vi "FTW-ProjectItemManager-Write-Session.vi"(0 "Project Item Manager":refnum<class "FTW-ProjectItemManager.lvclass">, 5 "Tag":string, 7 "Value":variant, 11 "error in":errorcluster) -> (4 "Project Item Manager out":refnum<class "FTW-ProjectItemManager.lvclass">, 15 "error out":errorcluster)   [LabVIEW 2012, in "FTW-ProjectItemManager.lvclass"]
doc: "This VI bypasses the Transaction Queue by writing a property directly to the Deploy Build Spec Project Item. The property is then persisted to disk if the user saves the LVProj, or if it is programmatically saved."
uses:
  FTW-ProjectItemManager.lvclass
  FTW-ProjectItemManager.lvclass/FTW-ProjectItemManager.ctl
panel:
  # "Inputs"
  # "Outputs"
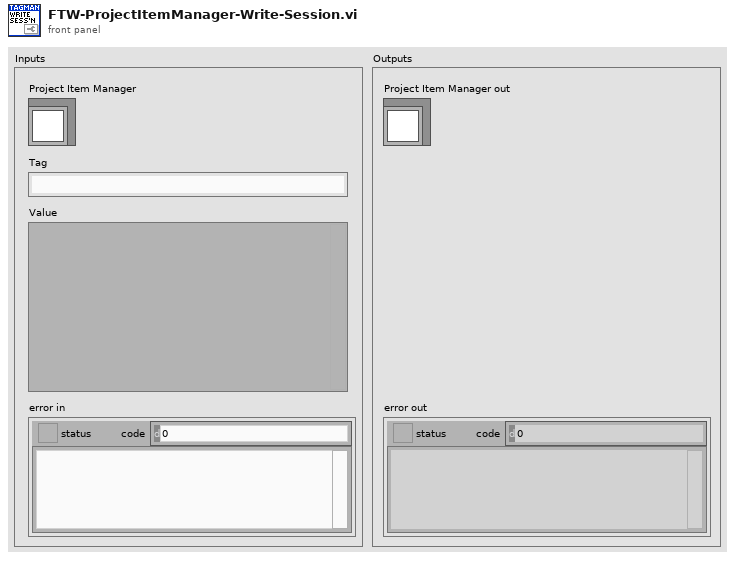
[diagram p1: front panel]
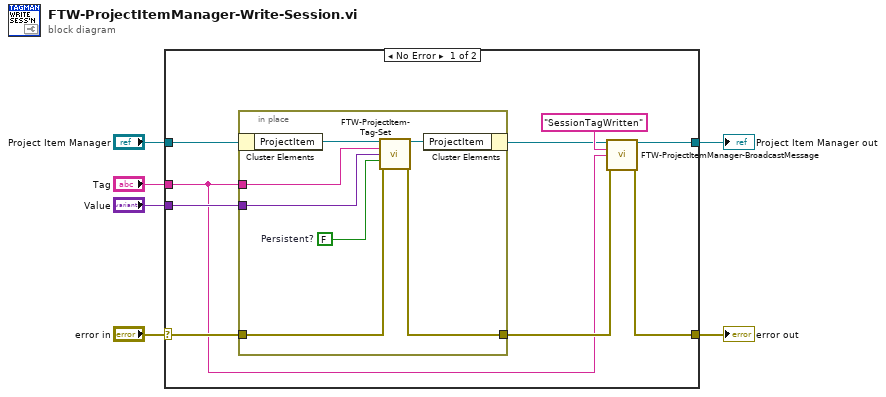
[diagram p0: block diagram]
diagram:
  n1 = case shown="No Error" "error in" {
    selector: "error in" -> [w14 w24]
    tunnel: [w11 w24] -> w6
    tunnel: [w12 w23] -> w4
    tunnel: "Project Item Manager" -> [w8 w23]
    tunnel: "Tag" -> [w9 _]
    tunnel: "Value" -> [w15 _]
    frame No Error {
      n2 = in-place {
        in-place-border: w15 -> [w22]
        in-place-border: w14 -> [w21]
        in-place-border: [w20] -> w10
        in-place-border: w9 -> [w19]
        w18 = FALSE  # Persistent?
        n3 = in-place-cluster #1(w8) -> ("ProjectItem"=w17:refnum<vi>)
        n4 = call "FTW-ProjectItem-Tag-Set.vi"("ProjectItem"=w17, "Tag Name"=w19, "Tag Value"=w22, "Persistent?"=w18, "error in"=w21) -> ("ProjectItem out"=w16:refnum<vi>, "error out"=w20:errorcluster)  [unwired: 9 in]
        n5 = in-place-cluster #1("ProjectItem"=w16) -> (w7:refnum<class "FTW-ProjectItemManager.lvclass">)
      }
      n6 = call "FTW-ProjectItemManager-BroadcastMessage.vi"("Project Item Manager"=w7, "Action Performed"="SessionTagWritten", "Payload"=w9, "error in"=w10) -> ("Project Item Manager out"=w12:refnum<class "FTW-ProjectItemManager.lvclass">, "error out"=w11:errorcluster)  [unwired: 10 in]
    }
    frame Error {
    }
  }
  "error out" <- w6
  "Project Item Manager out" <- w4
